vi "CreateSelfReference.vi"(8 "error in (no error)":errorcluster, 11 "SMO":refnum<class "SMO.lvclass">) -> (0 "error out":errorcluster, 3 "SMO out":refnum<class "SMO.lvclass">)   [LabVIEW 2013, in "SMO.lvclass"]
uses:
  SMO.lvclass
  SMO.lvclass/SMO.ctl
panel:
  # "For instructions on how to use the JKI State Machine Objects, examples and video tutorials, visit:\nhttp://jki.net/state-machine-objects/\n\nJKI State Machine Objects™\nhttp://jki.net/state-machine-objects/\nCopyright (C) 2005-2015, JKI <info@jki.net>\nALL RIGHTS RESERVED"
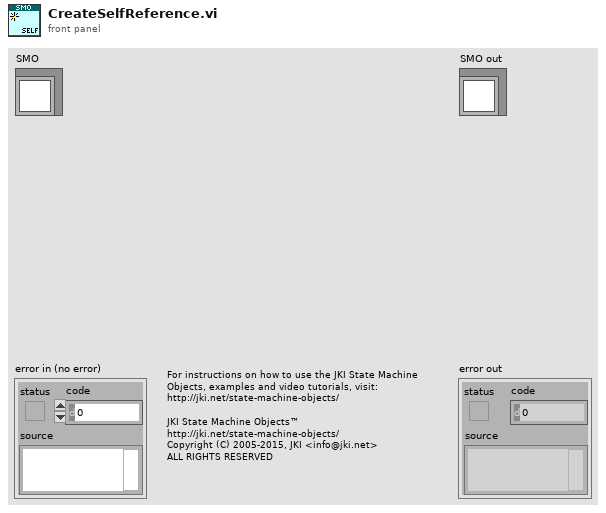
[diagram p1: front panel]
types:
  T1 = typedef "SMO.lvclass/PrivateData--Ref.ctl" = refnum<data-value>
  T2 = typedef "SMO.lvclass/PrivateData--Cluster.ctl" = cluster{"SMO Name":string, "Parent Call":T3, "Registered Processes":T4[], "Process Sync RendezVous":T5, "Process Error Notifier":refnum<notifier>, "Protected Events":T6, "Public Events":T7}
  T3 = typedef "SMO.lvclass/Parent Call--Enum.ctl" = enum16{"Allows parent to run", "Does not request parent to run"}
  T4 = typedef "SMO.lvclass/RegisteredProcessData--Cluster.ctl" = cluster{"Name":string, "Static VI Ref":refnum<vi>, "Running":bool}
  T5 = typedef "Rendezvous RefNum" = refnum<k1>
  T6 = typedef "SMO.lvclass/Protected Events.ctl" = cluster{"StopProcesses":refnum<user-event>, "AbortProcesses":refnum<user-event>}
  T7 = typedef "SMO.lvclass/Public Events.ctl" = cluster{"Error":refnum<user-event>}
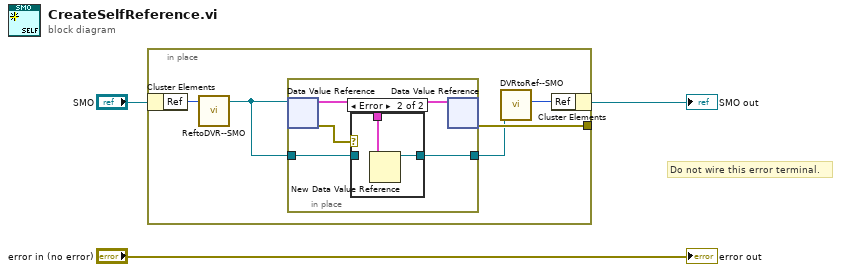
[diagram p0: block diagram]
diagram:
  # "Do not wire this error terminal."
  n1 = in-place {
    in-place-border: [w8] -> _
    n2 = in-place-cluster #1("SMO") -> ("Ref"=w7:u32)
    n3 = call "ReftoDVR--SMO.vi"("Ref"=w7) -> ("Ref"=w6:T1)  [unwired: 10 in]
    n4 = in-place {
      in-place-border: [w12] -> w5
      in-place-border: w6 -> [w9]
      n5 = in-place-dvr #2(w6) -> (w11:T2, w10:errorcluster)
      n6 = case shown="Error" w10 {
        tunnel: [w13 w15] -> w12
        tunnel: w11 -> [_ w14]
        tunnel: w9 -> [w13 _]
        frame No Error {
        }
        frame Error {
          n7 = New Data Value Reference(data value=w14) -> (data value reference=w15:refnum<data-value>)  [unwired: 1 in, 1 out]
        }
      }
      n8 = in-place-dvr #2(w11) -> (w8:errorcluster)  [unwired: 1 out]
    }
    n9 = call "DVRtoRef--SMO.vi"("Ref"=w5) -> ("Ref"=w4:u32)  [unwired: 10 in]
    n10 = in-place-cluster #1("Ref"=w4) -> (→"SMO out":refnum<class "SMO.lvclass">)
  }
  "error out" <- "error in (no error)"
